vi "Class Arr to Tree Arr.vi"(11 "Sorted Classes":T1(array[cluster])) -> (3 "Array":T2(array[cluster]))   [LabVIEW 2023]
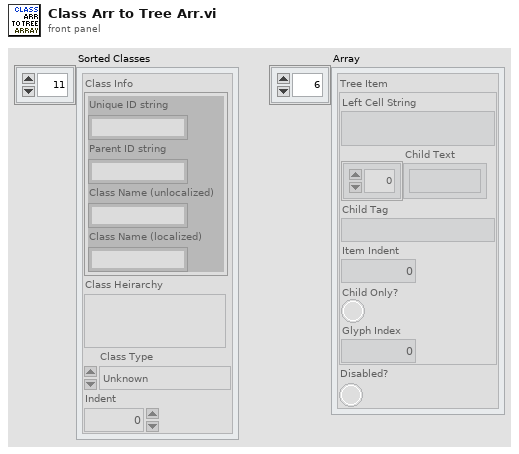
[diagram p1: front panel]
types:
  T1 = cluster{"Class Info":cluster{"Unique ID string":string, "Parent ID string":string, "Class Name (unlocalized)":string, "Class Name (localized)":string}, "Class Heirarchy":string, "Class Type":enum16{"Unknown", "Base", "Scripting", "Private", "Deprecated", "None", "Divider"}, "Indent":u32}[]
  T2 = cluster{"Tree Item":cluster{"Left Cell String":string, "Child Text":string[], "Child Tag":string, "Item Indent":i32, "Child Only?":bool, "Glyph Index":i32}, "Disabled?":bool}[]
  T3 = cluster{"Tree Item":cluster{"Left Cell String":string, "Child Text":string[], "Child Tag":string, "Item Indent":i32, "Child Only?":bool, "Glyph Index":i32}, "Disabled?":bool}
  T4 = enum16{"[NONE]", "Wire Bundle", "Wire Unbundle", "Terminal Unbundle", "Terminal Bundle", "Bundler Insert", "Bundler Remove", "Bundler Rearrange", "In Place Insert", "In Place Remove", "In Place Rearrange", "Wire Properties", "Wire Method", "Terminal Properties", "Terminal Method", "Properties Insert", "Properties Remove", "Properties Rearrange", "Method Change", "Classes"}
  T5 = enum16{"Unknown", "Base", "Scripting", "Private", "Deprecated", "None", "Divider"}
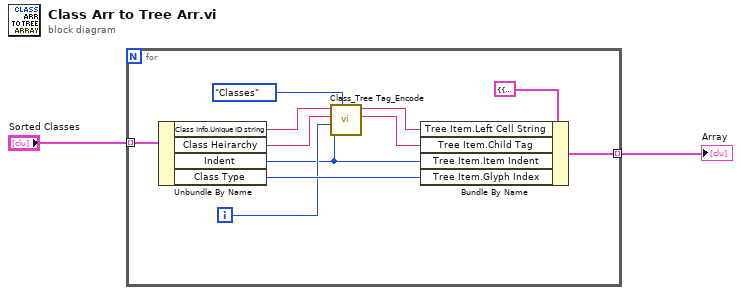
[diagram p0: block diagram]
diagram:
  n1 = for {
    tunnel: "Sorted Classes" -> [w12] mode=indexing
    tunnel: [w13] -> w2 mode=indexing
    i -> [w6]
    n2 = Unbundle By Name(w12) -> ("Class Info.Unique ID string"=w9:string, "Class Heirarchy"=w8:string, "Indent"=w5:u32, "Class Type"=w11:T5)
    n3 = call "Class_Tree Tag_Encode.vi"("Action"=T4."Classes", "Property Type"=w5, "Index"=w6, "Hierarchy"=w8, "Unique ID string"=w9) -> ("Tag"=w3:string, "Display name"=w4:string)  [unwired: 3 in, 2 out]
    n4 = Bundle By Name(cluster=T3 {"Tree Item"={"Left Cell String"="", "Child Text"=[], "Child Tag"="", "Item Indent"=0, "Child Only?"=FALSE, "Glyph Index"=0}, "Disabled?"=FALSE} ("Property For Tree with Disabled"), "Tree Item.Left Cell String"=w4, "Tree Item.Child Tag"=w3, "Tree Item.Item Indent"=w5, "Tree Item.Glyph Index"=w11) -> (w13:T3)
  }
  "Array" <- w2
